vi "_GroupAttributeValue.vi"(2 "error in":errorcluster, 3 "attribute value":T2={"device name"="", "attribute name"="", "quality value"=0, "quality string"="", "timestamp"=0.0, "dim. x"=0, "dim. y"=0, "value"=[], "error code"=0, "error stack"=[], "data type"=36}, 4 "attribute name":string, 5 "group id":i32) -> (0 "error out":errorcluster, 1 "attributes_values":T1(array[cluster]))   [LabVIEW 2014, in "tango.lvlib"]
uses:
  tango.lvlib
  tango_binding.so
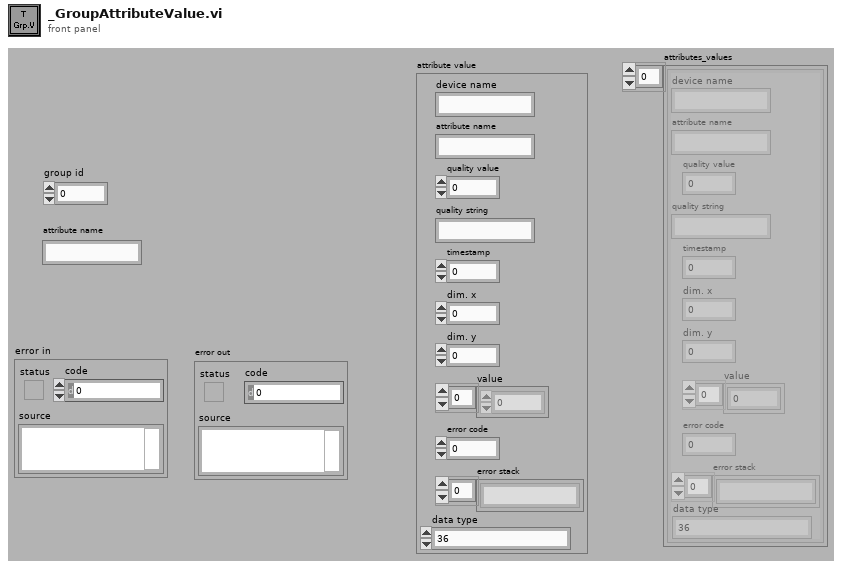
[diagram p1: front panel]
types:
  T1 = cluster{"device name":string, "attribute name":string, "quality value":i16, "quality string":string, "timestamp":dbl, "dim. x":i32, "dim. y":i32, "value":u8[], "error code":i32, "error stack":string[], "data type":u16}[]
  T2 = cluster{"device name":string, "attribute name":string, "quality value":i16, "quality string":string, "timestamp":dbl, "dim. x":i32, "dim. y":i32, "value":u8[], "error code":i32, "error stack":string[], "data type":u16}
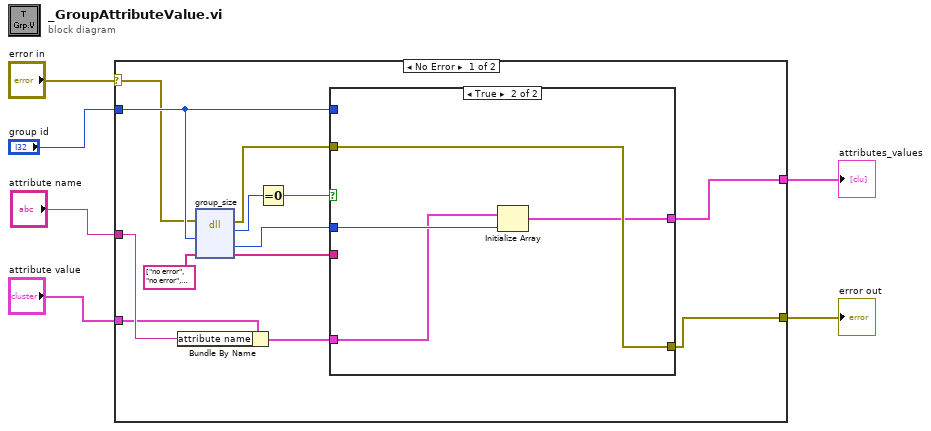
[diagram p0: block diagram]
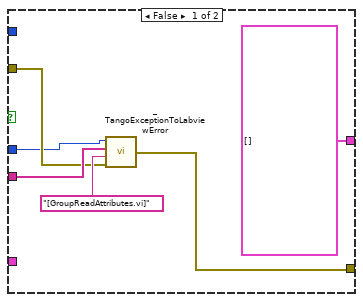
[diagram p2: hidden frame]
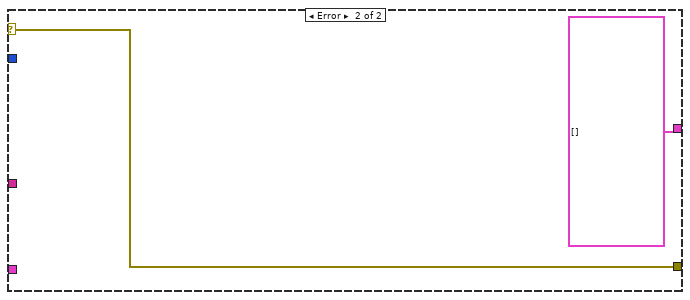
[diagram p3: hidden frame]
diagram:
  n1 = case shown="No Error" "error in" {
    selector: "error in" -> [w13 w31]
    tunnel: "group id" -> [w19 _]
    tunnel: "attribute name" -> [w10 _]
    tunnel: [w7 T1 []] -> w1
    tunnel: [w11 w31] -> w6
    tunnel: "attribute value" -> [w9 _]
    frame No Error {
      n2 = Bundle By Name(cluster=w9, "attribute name"=w10) -> (w8:T2)
      n3 = dll-call lib="tango_binding.*" fn="group_size"(error in=w13, "group_id"=w19, "error_stack"=string[] ["no error", "no error", "no error", "group_size"] ("error stack")) -> (error out=w12:errorcluster, "type de retour"=w14:i32, "size"=w17:i32, "error_stack"=w15:string[])  [unwired: 4 in, 1 out]
      n4 = Equal To 0?(x=w14) -> (x = 0?=w16:bool)
      n5 = case shown="True" w16 {
        tunnel: w19 -> [_ _]
        tunnel: w17 -> [w20 w29]
        tunnel: w15 -> [w23 _]
        tunnel: [w25 w28] -> w11
        tunnel: w12 -> [w21 w28]
        tunnel: [T1 [] w26] -> w7
        tunnel: w8 -> [_ w27]
        frame False {
          n6 = call "_TangoExceptionToLabviewError.vi"("error in"=w21, "location"="[GroupReadAttributes.vi]", "error stack"=w23, "error code"=w20) -> ("error out"=w25:errorcluster)
        }
        frame True {
          n7 = Initialize Array(w27, w29) -> (w26:T1)
        }
      }
    }
    frame Error {
    }
  }
  "error out" <- w6
  "attributes_values" <- w1
